vi "MainTmayra.vi"() -> ()   [LabVIEW 2019]
panel:
  out "time between obtaining data (ms)":u32
  in  "Tab Control":enum32{"Pressure", "Temperature"}(tab)
  out "Waveform Chart 2":cluster{dbl, dbl, dbl}(graph)
  in  "VISA resource name":refnum<visa-resource-name>="COM3"
  in  "termination char\n(0xA = '\\n' = LF)":u8=13 format="%.0x"
  in  "Recieve Data":bool
  out "Waveform Chart":T1(graph)
  in  "physical channels":tag="PXI1Slot2/ai2"
  in  "resistance configuration":i32(ring)=2 items=["2-Wire"=2, "3-Wire"=3, "4-Wire"=4]
  out "data":dbl[](array[numeric]) format="%0.2f"
  in  "stop program":bool
  # "NEGRO"
  # "bateria"
  # "BLANCO platina"
  # "VERDE fuente"
  # "AZUL MCU"
  # "AMARILLO AMBIENTE"
  # "ROJO BATERIA RELOJ"
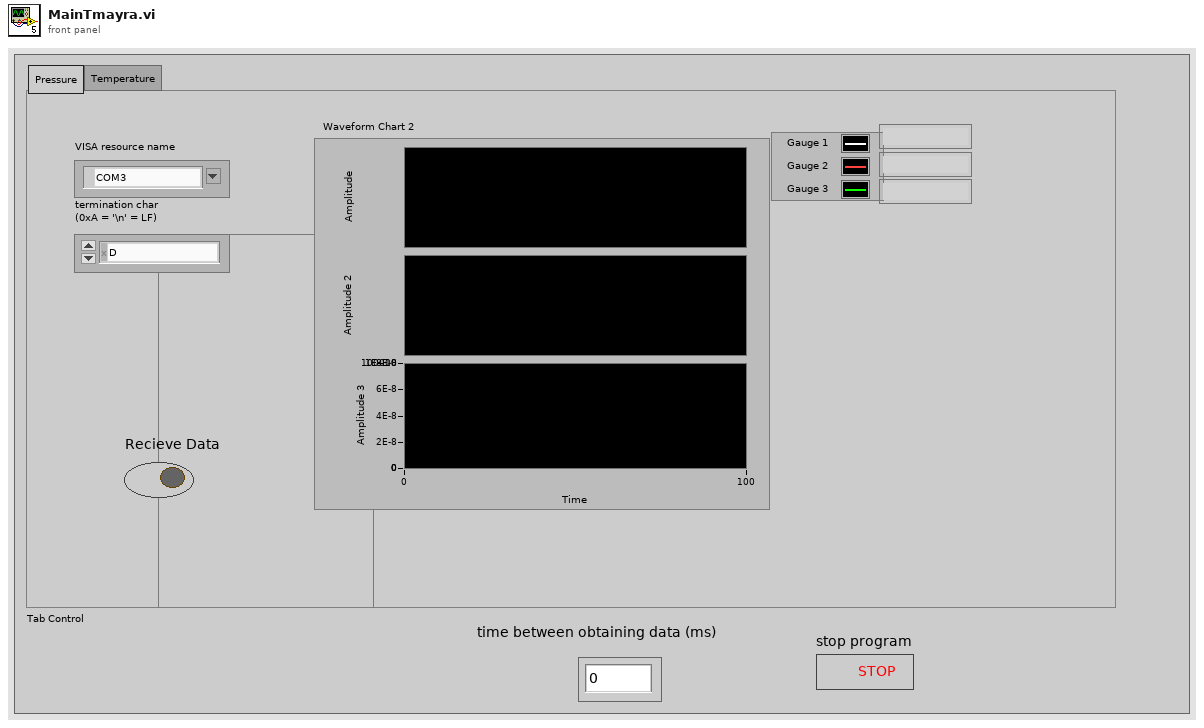
[diagram p1: front panel]
types:
  T1 = cluster{"data[0]":dbl, "data[1]":dbl, "data[2]":dbl, "data[3]":dbl, "data[4]":dbl, "data[5]":dbl, "data[6]":dbl, "data[7]":dbl, "data[8]":dbl, "data[9]":dbl, "data[10]":dbl, "data[11]":dbl, "data[12]":dbl, "data[13]":dbl, "data[14]":dbl, "data[15]":dbl, "data[16]":dbl, "data[17]":dbl, "data[18]":dbl, "data[19]":dbl}
  T2 = enum16{"open", "replace", "create", "open or create", "replace or create", "replace or create with confirmation"}
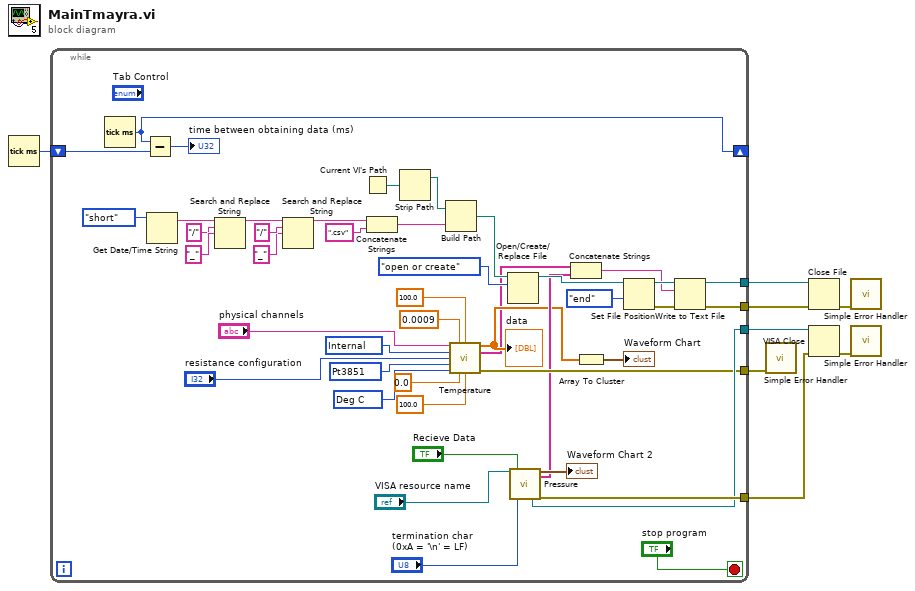
[diagram p0: block diagram]
diagram:
  n1 = Tick Count (ms)() -> (millisecond timer value=w1:u32)
  n2 = while {
    tunnel: [w48] -> w8
    tunnel: [w47] -> w7
    tunnel: [w46] -> w5
    tunnel: [w37] -> w3
    tunnel: [w36] -> w2
    shift-right: [w24] -> _
    shift-left: w1 -> [w23]
    stop <- "stop program" stop-if-true
    w30 = 10143 items=["Deg C"=10143, "Deg F"=10144, "Kelvins"=10325, "Deg R"=10145, "From Custom Scale"=10065] ("units")
    w31 = 10071 items=["Pt3750"=12481, "Pt3851"=10071, "Pt3911"=12482, "Pt3916"=10069, "Pt3920"=10053, "Pt3928"=12483, "Custom"=10137] ("rtd type")
    w32 = 10200 items=["Internal"=10200, "External"=10167, "None"=10230] ("current excitation source")
    n3 = Tick Count (ms)() -> (millisecond timer value=w24:u32)
    n4 = Subtract(x=w24, y=w23) -> (x-y=→"time between obtaining data (ms)":u32)
    n5 = Get Date/Time String(date format (0)=enum16{"short", "long", "abbreviated"}."short") -> (date string=w14:string)  [unwired: 2 in, 1 out]
    n6 = Search and Replace String(input string=w14, search string="/", replace string="_" ("replace string (\"\")")) -> (result string=w17:string)  [unwired: 5 in, 3 out]
    n7 = Search and Replace String(input string=w17, search string="/", replace string="_" ("replace string (\"\")")) -> (result string=w12:string)  [unwired: 5 in, 3 out]
    n8 = Current VI's Path() -> (path=w42:path)
    n9 = Concatenate Strings(w12, ".csv" ("string")) -> (w11:string)
    n10 = Strip Path(path=w42) -> (stripped path=w43:path)  [unwired: 1 out]
    n11 = Build Path(base path=w43, name or relative path=w11) -> (appended path=w44:path)
    n12 = call "Temperature.vi"("physical channels"="physical channels", "current excitation value"=0.0009, "r0"=100.0, "current excitation source"=w32, "resistance configuration"="resistance configuration", "rtd type"=w31, "units"=w30, "minimum value"=0.0, "maximum value"=100.0) -> ("data"=w20:dbl[], "output array"=w9:string[], "error out"=w46:errorcluster)  [unwired: 4 in]
    "data" <- w20
    n13 = Open/Create/Replace File(file path (use dialog)=w44, operation (0:open)=T2."open or create") -> (refnum out=w45:refnum<file>)  [unwired: 4 in, 2 out]
    n14 = call "Pressure.vi"("VISA resource name"="VISA resource name", "Recieve Data"="Recieve Data", "termination char\n(0xA = '\\n' = LF)"="termination char\n(0xA = '\\n' = LF)") -> ("VISA resource name out"=w47:refnum<visa-resource-name>, "output cluster"=→"Waveform Chart 2":cluster{dbl, dbl, dbl}, "output array"=w21:string[], "error out"=w48:errorcluster)  [unwired: 10 in, 3 out]
    n15 = Concatenate Strings(w9, w21) -> (w22:string)
    n16 = Array To Cluster(array=w20) -> (cluster=→"Waveform Chart":T1)
    n17 = Set File Position(refnum=w45, from (0:start)=enum16{"start", "end", "current"}."end") -> (refnum out=w39:refnum<file>, error out=w38:errorcluster)  [unwired: 2 in]
    n18 = Write to Text File(file (use dialog)=w39, text=w22, error in=w38) -> (refnum out=w37:refnum<file>, error out=w36:errorcluster)  [unwired: 1 in, 1 out]
  }
  n19 = call <vilib>:"Simple Error Handler.vi"("error in (no error)"=w5) -> ()  [unwired: 4 in, 5 out]
  n20 = Close File(refnum=w3, error in=w2) -> (error out=w4:errorcluster)  [unwired: 1 out]
  n21 = VISA Close(VISA resource name=w7, error in (no error)=w8) -> (error out=w6:errorcluster)
  n22 = call <vilib>:"Simple Error Handler.vi"("error in (no error)"=w4) -> ()  [unwired: 1 in, 8 out]
  n23 = call <vilib>:"Simple Error Handler.vi"("error in (no error)"=w6) -> ()  [unwired: 4 in, 5 out]
